vi "atten.vi"() -> ()   [LabVIEW 2017]
panel:
  out "PS":dbl
  out "i":i32
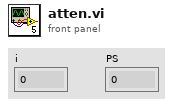
[diagram p1: front panel]
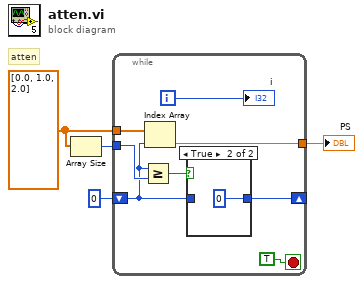
[diagram p0: block diagram]
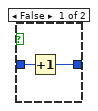
[diagram p2: hidden frame]
diagram:
  w4 = dbl[] [0.0, 1.0, 2.0]
  # "atten"
  n1 = Array Size(array=w4) -> (size(s)=w1:i32)
  n2 = while {
    shift-right: [w10] -> _
    shift-left: 0 -> [w9]
    tunnel: w4 -> [w8]
    tunnel: w1 -> [w11]
    tunnel: [w7] -> w2
    i -> [w12]
    stop <- TRUE stop-if-true
    n3 = Greater Or Equal?(x=w9, y=w11) -> (x >= y?=w5:bool)
    n4 = Index Array(array=w8, index=w9) -> (element=w7:dbl)
    n5 = case shown="True" w5 {
      tunnel: [w14 0] -> w10
      tunnel: w9 -> [w13 _]
      frame False {
        n6 = Increment(x=w13) -> (x+1=w14:i32)
      }
      frame True {
      }
    }
    "i" <- w12
  }
  "PS" <- w2
